vi "AlliGator Build Dataset Information String.vi"() -> (3 "Dataset Information String":string)   [LabVIEW 2021, in "AlliGator Dataset Information Window.lvlib"]
doc: "Creates <B>Dataset Information String</B> based on internal variables and settings."
uses:
  AlliGator Dataset Information Window.lvlib
  Globals, Variables, Constants/AlliGator Variables List.ctl
  Settings/AlliGator Settings List.ctl
  Variant/Variant to Data/Variant to String.vi
  Variant/Variant to Data/Variant to I32.vi
  Variant/Variant to Data/Variant to Boolean.vi
  Variant/Variant to Data/Variant to Path.vi
  Globals, Variables, Constants/AlliGator Globals, Variables & Constants.lvlib
  Variant/Variant to Data/Variant to Data.lvlib
  Settings/AlliGator Settings.lvlib
  Files/AlliGator Files.lvlib
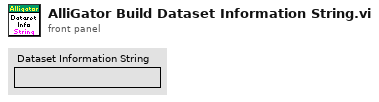
[diagram p1: front panel]
types:
  T1 = typedef "AlliGator Globals, Variables & Constants.lvlib/AlliGator Variables List.ctl" = enum16{"---- GUI ----", "GUI:Initialization Status", "GUI:State Indicators Refnum", "GUI:Original AlliGator Menu Items", "GUI:Current Action Loop State", "GUI:Script in progress", "GUI:Playback", "GUI:Loop Playback", "GUI:Search ROI Used", "GUI:Search ROI", "Decay Graph Max Legend Size", "Intensity Graph Max Legend Size", "Decay Statistics Graph Max Legend Size", "Phasor Graph Max Legend Size", "Phasor Ratio Graph Max Legend Size", "Lifetime Graph Max Legend Size", "---- Files ----", "Files:Export Dataset Frames as Individual Files", "Files:Show Batch Export Help Balloons", "Files:Frames in Dataset", "Files:ptu File Frame Start Indices", "Files:Current Frame in Dataset", "Files:Current Frame Timestamp", "Files:Dataset Loaded", "Files:Dataset Metadata", "Files:Dataset Channel", "Files:Dataset Data Description", "Files:Background Dataset Metadata", "Files:Background Dataset Channel", "Files:Background Dataset Data Description", "Files:Background File Subtraction", "Files:Background File Path", "Files:Background File Pile-up Correction", "Files:Background File Pixel Well Capacity", "Files:Background File Scaling Factor", "Files:Current Dataset Load Settings", "Files:Dataset Path", "Files:ICCD-specific Information", "Files:Macrotime Gate Separation", "------ Python Plugins ------", "Python Plugins:Information", "Python Plugins:Python Session", "Python Plugins:Valid Python Session?", "---- Source Image ----", "Source Image:ROIs", "Source Image:Current ROI", "Source Image:ROI Event Refnum", "X_Source Image Display Range", "X_Source Image Palette Information", "X_Type of Displayed Image", "X_Time Gate Slider", "Source Image:Palette List", "Source Image:Scale", "Source Image:ROI Overlay Color", "Source Image:Overlay to Erase", "Source Image:Is Displayed Image Accumulated", "Source Image:White Light Image Modified", "Source Image:Mask Image Modified", "---- Image Profile Window ----", "Image Profile:Window Event Refnum", "Image Profile:IntensityType", "Image Profile:Intensity Average Type", "Image Profile:Intensity-weighted SDV", "Image Profile:Box Profile Type", "Image Profile:Window Open", "Image Profile:Plotted Fit Parameter", "------ Phasor Graph -------", "Phasor Graph:Show Line", "---- Phasor Plot ---", "Phasor Plot:Parameters Changed", "Phasor Plot:FLI Dataset Modified since last Calculation", "Phasor Harmonics Data", "Selected Phasor Harmonics", "Phasor Harmonic Manager Event Refnum", "Phasor Plot:ROIs", "Phasor Plot:Current ROI", "Phasor Plot:ROI Event Refnum", "Phasor Plot:Image Reference Points", "Phasor Plot:Computed", "Phasor Plot:Palette Information", "Phasor Plot:Palette List", "Phasor Plot:Phasor Ratio Palette Information", "Phasor Plot:Phasor Ratio Palette List", "Phasor Plot:Image Scale", "Phasor Plot:Image Overlay to Erase", "Phasor Plot:Image Elements to Update", "Phasor Plot:Current Calculation Parameters", "Phasor Plot:Current Calibration Options", "Phasor Plot:Reset Cumulated Phasor Plot", "Phasor Plot:Reference 1", "Phasor Plot:Lifetime Reference 1", "Phasor Plot:Reference 1 Frequency", "Phasor Plot:Reference 2", "Phasor Plot:Lifetime Reference 2", "Phasor Plot:Reference 2 Frequency", "---- Decay Analysis ----", "Number of Selected Decays to Fit", "LS Fit Results", "LAR Fit Results", "BS Fit Results", "Last Decay Max - Min", "Best Fit Parameters", "Best Fit Parameter Names", "Actual Size X", "Actual Size Y", "Binning X", "Binning Y", "Actual # Gates", "Dataset Number", "Gates to...", "Gates Skipped", "Gates to keep", "Gate Step", "Gate Separation", "Reversed Gates", "Pile-up Correction", "Pixel Well Capacity", "Background Subtracted", "Background Subtraction Method", "Background Definition Range", "Background File (deprecated)", "Number of Dataset Accumulated", "Array of Accumulated Dataset Paths", "Do Averaged Datasets", "Destination File Path", "Process Plot Target", "Use 1/D as Phasor Frequency", "---- Decay Fit Parameter Map -----", "Decay Fit Parameter Map:Palette Information", "Decay Fit Parameter Map:Palette List", "---- Parameter Map ----", "Parameter Map:Palette Information", "Parameter Map:Palette List", "------- Local Decay Window ---------", "Local Decay Graph Window:Event Refnum", "Local Decay Graph Window:Use normalized IRF for convolution", "----- Miscellaneous ----", "Misc:Skippable Dialog Windows Status"}
  T2 = typedef "AlliGator Settings.lvlib/AlliGator Settings List.ctl" = enum16{"GUI:Visible Settings Tab", "GUI:Last Run Version", "Source Image:Use Image Histogram for Contrast", "Source Image:Low Count Pixels Rejection Options", "Source Image:High Count Pixels Rejection Options", "Source Image:Use Image Brightness", "Source Image:Blend Overlay with Image Background", "Source Image:Use Fixed ROI Diameter", "Source Image:ROI Diameter", "Source Image:ROI Center Color", "Source Image:Peak Threshold", "Source Image:Intensity Threshold", "Source Image:Image Binning Options", "Source Image:Image Smoothing Options", "Source Image:Image Histogram Active", "Source Image:Invert Binary Mask", "Source Image:Hot Pixel Removal", "Source Image:Overlay Analyzed ROI Center", "Source Image:Auto-Adjust Contrast", "Source Image:Histogram Lower Percentile", "Source Image:Histogram Upper Percentile", "Source Image:Save Source Image", "Source Image:Scale Bar Options", "Source Image:Image Resolution (Pixel Size)", "Source Image:Flatfield Correction", "Source Image:Show Dead Left Columns Correction", "Source Image:Dead Left Columns Correction", "Source Image:Image Pre-Processing Operations Order", "Source Image:Overlay ROI Median", "Source Image:Median Overlay Color", "Data Information:Gate Width", "Data Information:Nanotime Gate Separation", "Data Information:Macrotime Gate Separation", "Data Information:Gate Step", "Data Information:# Gates", "Data Information:Gate Image Exposure", "Data Information:Gate Image Integration", "Data Information:Gates to Skip", "Data Information:Gates to Keep", "Data Information:Define Gates to", "Data Information:Channel Name", "Data Information:Available Channel Names", "Data Information:Channel Arithmetic", "Data Information:Background File Subtraction", "Data Information:Background File", "Data Information:Background Scaling Factor", "Data Information:Background Pile-up Correction", "Data Information:Background Pixel Well Capacity", "Data Information:Laser Period", "Data Information:SYNC Period", "Data Information:Pile-up Correction", "Data Information:Pixel Well Capacity", "Data Information:Dataset Scaling Factor", "Fluorescence Decay_Decay Pre-Processing:Reverse Gates", "Fluorescence Decay_Decay Pre-Processing:Verbose Decay Pre-Processing", "Fluorescence Decay_Decay Pre-Processing:Use Decay Pre-Processing", "Fluorescence Decay_Decay Pre-Processing:Background Subtraction", "Fluorescence Decay_Decay Pre-Processing:Background Definition Range", "Fluorescence Decay_Decay Pre-Processing:Baseline Subtraction Method", "Fluorescence Decay_Decay Pre-Processing:Decay Pre-Processing Operations Order", "Fluorescence Decay_Decay Pre-Processing:Smoothing Parameter", "Fluorescence Decay_Decay Pre-Processing:Shift Decay", "Fluorescence Decay_Decay Pre-Processing:Decay Shift Parameters", "Fluorescence Decay_Decay Pre-Processing:Fold Decay", "Fluorescence Decay_Decay Pre-Processing:# Folds", "Fluorescence Decay_Decay Pre-Processing:1-Normalize Decay", "Fluorescence Decay_Decay Pre-Processing:[0-1]-Normalize Decay", "Fluorescence Decay_Decay Pre-Processing:Smoothen Decay", "Fluorescence Decay_Decay Pre-Processing:Extrapolate Decay", "Fluorescence Decay_Decay Pre-Processing:Use Periodicity", "Fluorescence Decay_Decay Pre-Processing:Use Cursors", "Fluorescence Decay_Decay Pre-Processing:Tail Fraction", "Fluorescence Decay_Decay Pre-Processing:Head Fraction", "Fluorescence Decay_Decay Pre-Processing:Additional Points", "Fluorescence Decay_Decay Pre-Processing:Straighten Decay", "Fluorescence Decay_Decay Pre-Processing:Constant Background", "Fluorescence Decay_Decay Pre-Processing:Pixel-Normalize Decay", "Fluorescence Decay_Advanced Analysis:Extract IRF instead of Decay", "Fluorescence Decay_Advanced Analysis:IRF Extraction Options", "Fluorescence Decay_Advanced Analysis:IRF Optimization Options", "Fluorescence Decay_Advanced Analysis:Square Pulse Options", "Fluorescence Decay_Advanced Analysis:IRF Order", "Fluorescence Decay_Advanced Analysis:IRF Time Constants", "Fluorescence Decay_Advanced Analysis:Wavelet Analysis Options", "Fluorescence Decay_Advanced Analysis:Average Lifetime Options", "Fluorescence Decay_Fit Options:Fit Options", "Fluorescence Decay_Fit Options:Use Legacy Fitting Approach", "Fluorescence Decay_Fit Options:Use Data Information Laser Period", "Fluorescence Decay_Fit Parameters:Displayed Fit Parameters", "Fluorescence Decay_Fit Parameters:Fit Parameter Constraints", "Fluorescence Decay_Fit Parameters:Export Tabulated Results", "Fluorescence Decay_Fit Parameters:MLE Baseline Offset Type", "Fluorescence Decay_Fit Parameters:MLE Baseline Offset", "Fluorescence Decay_Fit Parameters:Guess Parameter Names", "Fluorescence Decay_Fit Parameters:Guess Parameter Values", "Fluorescence Decay_Fit Parameters:Guess Parameters Options", "Fluorescence Decay_Styles:Show Last Decay Only", "Fluorescence Decay_Styles:Decay Graph Color Array", "Fluorescence Decay:Decay Graph Active", "Fluorescence Decay Statistics:Min Peak Value", "Fluorescence Decay Statistics:Reject Low Decay Peak Pixels", "Fluorescence Decay Statistics:Reject High Decay Peak Pixels", "Fluorescence Decay Statistics:Max Peak Value", "Time Traces:Use File Timestamp", "Time Traces:Time Step", "Time Traces:Use Intensity Correction File", "Time Traces:Intensity Correction File", "Phasor Plot:Phasor Plot Smoothing Options", "Phasor Plot:Phasor Plot Size", "Phasor Plot:Phasor Plot Graphics Options", "Phasor Plot:Cumulative Phasor Plot", "Phasor Plot:Use Phasor Brightness", "Phasor Plot:Blend Overlay with Phasor Background", "Phasor Plot:Save Phasor Plot", "Phasor Plot:Show References", "Phasor Plot:Phasor Ratio Decay Range", "Phasor Plot:Exponential Fading", "Phasor Plot:Phasor Ratio Reference Colors", "Phasor Plot:Reference Radius", "Phasor Plot:Show Color Map Vertices", "Phasor Plot:Phasor Plot Active", "Phasor Plot:Phasor Ratio Color Map Type", "Phasor Plot:Phasor Ratio Color Map", "Phasor Plot:Phasor Ratio Display Range", "Phasor Plot:Selected Image ROI(s)", "Phasor Plot:All Image ROIs", "Phasor Plot:Selected Phasor Plot ROI(s)", "Phasor Plot:All Phasor Plot ROIs", "Phasor Plot:Phasor Ratio Color-Coded Quantity", "Phasor Plot:Store Phasor Harmonics", "Phasor Plot:Draw Reference Segment", "Phasor Plot:User-Defined Quantity", "Phasor Graph:Phasor Frequency", "Phasor Graph:Phasor Ratio Type", "Phasor Graph:Pixel-level Phasor Computation", "Phasor Graph:Save Phasor Graph", "Phasor Graph:Phasor Graph Active", "Phasor Graph:Phasor SDV Options", "Phasor Calibration:Use Backup Calibration if needed", "Phasor Graph:Define Shortest Lifetime as", "Phasor Calibration:Backup Calibration Type", "Phasor Calibration:Calibration Type", "Phasor Calibration:Calibration Lifetime", "Phasor Calibration:Calibration Map Algorithm", "Single-Exponential Phasor Locus (SEPL):Gate Parameters", "Single-Exponential Phasor Locus (SEPL):User-defined Gate", "Single-Exponential Phasor Locus (SEPL):User-defined IRF", "Single-Exponential Phasor Locus (SEPL):Phasor Parameters", "Single-Exponential Phasor Locus (SEPL):Decay & IRF Parameters", "Single-Exponential Phasor Locus (SEPL):Display Parameters", "Lifetime Analysis:Decay Analysis Parameters", "Lifetime Analysis:Lifetime Map Active", "Plugins:Python Settings", "Miscellaneous:Verbose Mode", "Miscellaneous:Beep after Script", "Miscellaneous:Saved Image File Format", "Miscellaneous:Exported Gate Image Settings", "Miscellaneous:Include Loading in Timing", "Miscellaneous:Verbose Settings Mode", "Miscellaneous:Histogram Options", "Miscellaneous:Beep on Error", "Miscellaneous:# Logical Processors Used", "Miscellaneous:ROI Description Max Characters", "Miscellaneous:Verbose Error Mode", "Miscellaneous:Transparent Mask Color"}
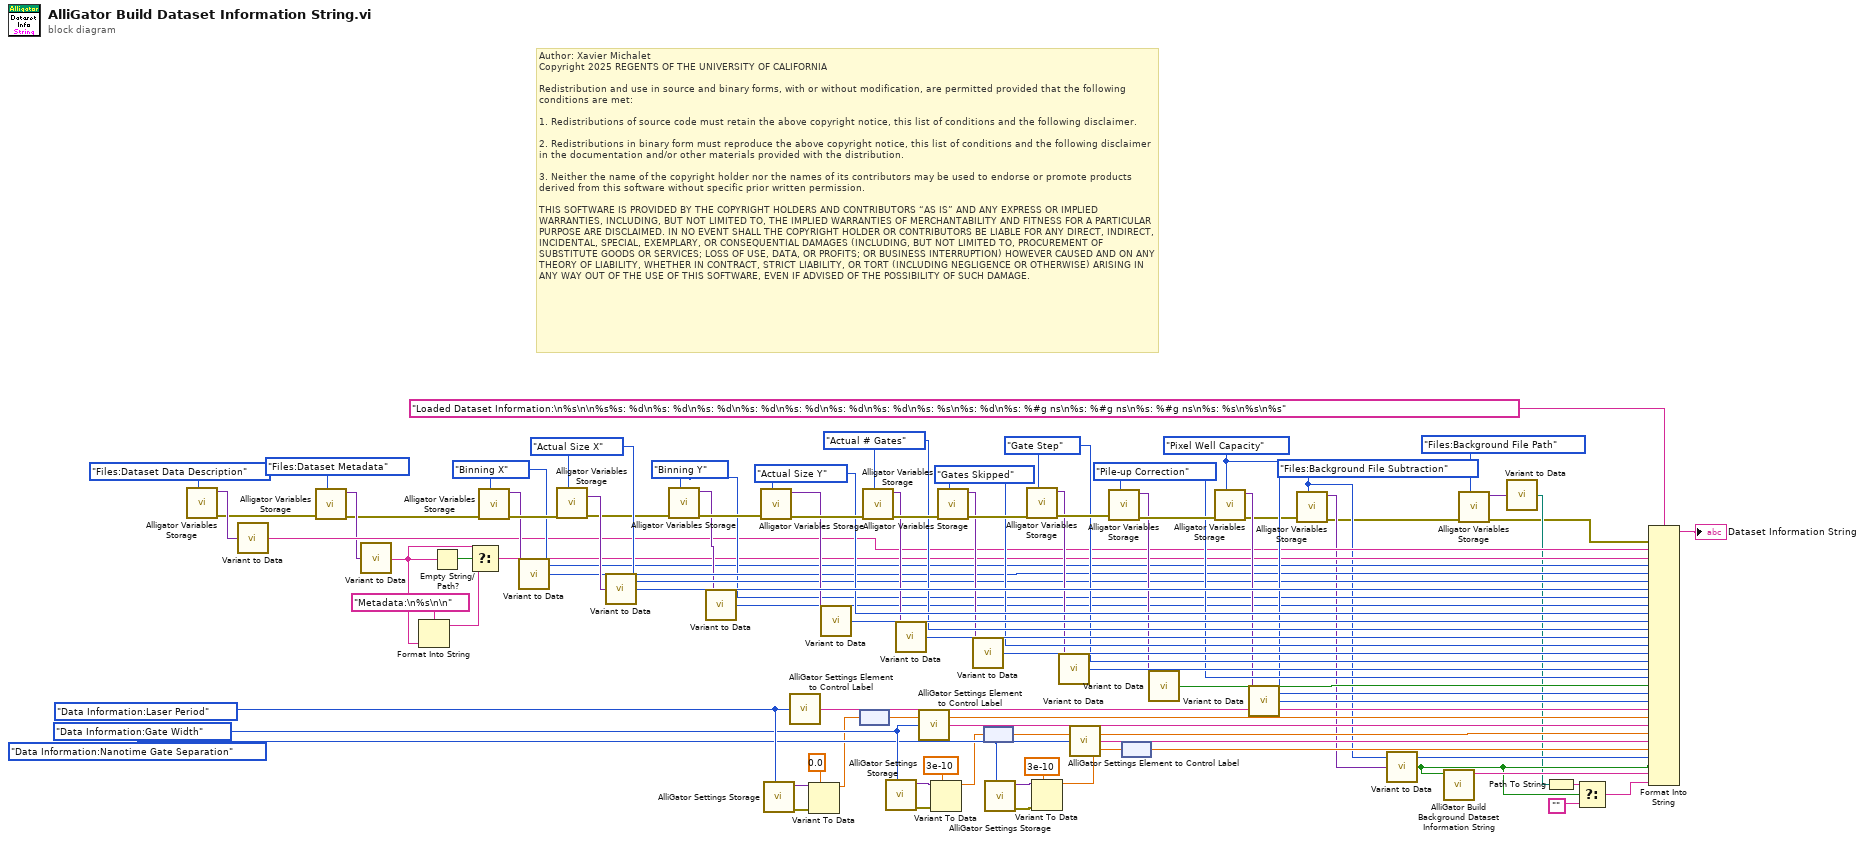
[diagram p0: block diagram]
diagram:
  w12 = AlliGator_Variables_List."Files:Background File Subtraction" ("Alligator Variable")
  w27 = AlliGator_Variables_List."Binning Y" ("Alligator Variable")
  w24 = AlliGator_Variables_List."Binning X" ("Alligator Variable")
  w46 = AlliGator_Settings_List."Data Information:Gate Width" ("AlliGator Settings List")
  w47 = AlliGator_Settings_List."Data Information:Laser Period" ("AlliGator Settings List")
  w45 = AlliGator_Settings_List."Data Information:Nanotime Gate Separation" ("AlliGator Settings List")
  w63 = AlliGator_Variables_List."Gate Step" ("Alligator Variable")
  w66 = AlliGator_Variables_List."Gates Skipped" ("Alligator Variable")
  w57 = AlliGator_Variables_List."Pixel Well Capacity" ("Alligator Variable")
  w60 = AlliGator_Variables_List."Pile-up Correction" ("Alligator Variable")
  w69 = AlliGator_Variables_List."Actual # Gates" ("Alligator Variable")
  w72 = AlliGator_Variables_List."Actual Size Y" ("Alligator Variable")
  w32 = AlliGator_Variables_List."Actual Size X" ("Alligator Variable")
  # "Author: Xavier Michalet\nCopyright 2025 REGENTS OF THE UNIVERSITY OF CALIFORNIA\n\nRedistribution and use in source and binary forms, with or without modification, are permitted provided that the following conditions are met:\n\n1. Redistributions of source code must retain the above copyright notice, this list of conditions and the following disclaimer.\n\n2. Redistributions in binary form must reproduce the above copyright notice, this list of conditions and the following disclaimer in the documentation and/or other materials provided with the distribution.\n\n3. Neither the name of the copyright holder nor the names of its contributors may be used to endorse or promote products derived from this software without specific prior written permission.\n\nTHIS SOFTWARE IS PROVIDED BY THE COPYRIGHT HOLDERS AND CONTRIBUTORS “AS IS” AND ANY EXPRESS OR IMPLIED WARRANTIES, INCLUDING, BUT NOT LIMITED TO, THE IMPLIED WARRANTIES OF MERCHANTABILITY AND FITNESS FOR A PARTICULAR PURPOSE ARE DISCLAIMED. IN NO EVENT SHALL THE COPYRIGHT HOLDER OR CONTRIBUTORS BE LIABLE FOR ANY DIRECT, INDIRECT, INCIDENTAL, SPECIAL, EXEMPLARY, OR CONSEQUENTIAL DAMAGES (INCLUDING, BUT NOT LIMITED TO, PROCUREMENT OF SUBSTITUTE GOODS OR SERVICES; LOSS OF USE, DATA, OR PROFITS; OR BUSINESS INTERRUPTION) HOWEVER CAUSED AND ON ANY THEORY OF LIABILITY, WHETHER IN CONTRACT, STRICT LIABILITY, OR TORT (INCLUDING NEGLIGENCE OR OTHERWISE) ARISING IN ANY WAY OUT OF THE USE OF THIS SOFTWARE, EVEN IF ADVISED OF THE POSSIBILITY OF SUCH DAMAGE."
  n1 = call "Alligator Variables Storage.vi"("AlliGator Variable"=AlliGator_Variables_List."Files:Dataset Data Description" ("Alligator Variable")) -> ("Error Out"=w20:errorcluster, "Data out"=w82:variant)  [unwired: 8 in, 1 out]
  n2 = call-poly "Variant to Data.vi"("Variant"=w82) -> ("String"=w23:string)  [unwired: 8 in]
  n3 = call "Alligator Variables Storage.vi"("AlliGator Variable"=AlliGator_Variables_List."Files:Dataset Metadata" ("Alligator Variable"), "Error In"=w20) -> ("Error Out"=w19:errorcluster, "Data out"=w22:variant)  [unwired: 7 in, 1 out]
  n4 = call-poly "Variant to Data.vi"("Variant"=w22) -> ("String"=w15:string)  [unwired: 8 in]
  n5 = Format Into String(format string="Metadata:\n%s\n\n", w15) -> (resulting string=w16:string)  [unwired: 2 in, 1 out]
  n6 = Empty String/Path?(string/path=w15) -> (empty?=w18:bool)
  n7 = Select(t=w15, s=w18, f=w16) -> (s? t:f=w17:string)
  n8 = call "Alligator Variables Storage.vi"("AlliGator Variable"=w24, "Error In"=w19) -> ("Error Out"=w33:errorcluster, "Data out"=w31:variant)  [unwired: 7 in, 1 out]
  n9 = call-poly "Variant to Data.vi"("Variant"=w31) -> ("Value"=w30:i32)  [unwired: 8 in]
  n10 = call "Alligator Variables Storage.vi"("AlliGator Variable"=w32, "Error In"=w33) -> ("Error Out"=w29:errorcluster, "Data out"=w74:variant)  [unwired: 7 in, 1 out]
  n11 = call-poly "Variant to Data.vi"("Variant"=w74) -> ("Value"=w73:i32)  [unwired: 8 in]
  n12 = call "Alligator Variables Storage.vi"("AlliGator Variable"=w27, "Error In"=w29) -> ("Error Out"=w28:errorcluster, "Data out"=w26:variant)  [unwired: 7 in, 1 out]
  n13 = call-poly "Variant to Data.vi"("Variant"=w26) -> ("Value"=w25:i32)  [unwired: 8 in]
  n14 = call "Alligator Variables Storage.vi"("AlliGator Variable"=w72, "Error In"=w28) -> ("Error Out"=w76:errorcluster, "Data out"=w71:variant)  [unwired: 7 in, 1 out]
  n15 = call "AlliGator Settings Storage.vi"("AlliGator Settings List"=w47) -> ("Error Out"=w53:errorcluster, "Variant Data out"=w54:variant)  [unwired: 9 in]
  n16 = call "AlliGator Settings Element to Control Label.vi"("AlliGator Settings List"=w47) -> ("Label"=w43:string)  [unwired: 8 in]
  n17 = Variant To Data(error in=w53, type=dbl[unit] 0.0 ("Laser Period"), Variant=w54) -> (data=w42:dbl[unit])  [unwired: 1 out]
  n18 = call-poly "Variant to Data.vi"("Variant"=w71) -> ("Value"=w70:i32)  [unwired: 8 in]
  n19 = node(w42) -> (w41:dbl)
  n20 = call "Alligator Variables Storage.vi"("AlliGator Variable"=w69, "Error In"=w76) -> ("Error Out"=w78:errorcluster, "Data out"=w68:variant)  [unwired: 7 in, 1 out]
  n21 = call "AlliGator Settings Storage.vi"("AlliGator Settings List"=w46) -> ("Error Out"=w51:errorcluster, "Variant Data out"=w52:variant)  [unwired: 9 in]
  n22 = call-poly "Variant to Data.vi"("Variant"=w68) -> ("Value"=w67:i32)  [unwired: 8 in]
  n23 = call "AlliGator Settings Element to Control Label.vi"("AlliGator Settings List"=w46) -> ("Label"=w40:string)  [unwired: 8 in]
  n24 = Variant To Data(error in=w51, type=dbl[unit] 3e-10 ("Gate Duration"), Variant=w52) -> (data=w39:dbl[unit])  [unwired: 1 out]
  n25 = call "Alligator Variables Storage.vi"("AlliGator Variable"=w66, "Error In"=w78) -> ("Error Out"=w79:errorcluster, "Data out"=w65:variant)  [unwired: 7 in, 1 out]
  n26 = call-poly "Variant to Data.vi"("Variant"=w65) -> ("Value"=w64:i32)  [unwired: 8 in]
  n27 = node(w39) -> (w38:dbl)
  n28 = call "AlliGator Settings Storage.vi"("AlliGator Settings List"=w45) -> ("Error Out"=w49:errorcluster, "Variant Data out"=w50:variant)  [unwired: 9 in]
  n29 = call "Alligator Variables Storage.vi"("AlliGator Variable"=w63, "Error In"=w79) -> ("Error Out"=w80:errorcluster, "Data out"=w62:variant)  [unwired: 7 in, 1 out]
  n30 = Variant To Data(error in=w49, type=dbl[unit] 3e-10 ("Gate Duration"), Variant=w50) -> (data=w35:dbl[unit])  [unwired: 1 out]
  n31 = call-poly "Variant to Data.vi"("Variant"=w62) -> ("Value"=w61:i32)  [unwired: 8 in]
  n32 = call "AlliGator Settings Element to Control Label.vi"("AlliGator Settings List"=w45) -> ("Label"=w37:string)  [unwired: 8 in]
  n33 = call "Alligator Variables Storage.vi"("AlliGator Variable"=w60, "Error In"=w80) -> ("Error Out"=w77:errorcluster, "Data out"=w59:variant)  [unwired: 7 in, 1 out]
  n34 = node(w35) -> (w34:dbl)
  n35 = call-poly "Variant to Data.vi"("Variant"=w59) -> ("Value"=w58:bool)  [unwired: 8 in]
  n36 = call "Alligator Variables Storage.vi"("AlliGator Variable"=w57, "Error In"=w77) -> ("Error Out"=w13:errorcluster, "Data out"=w55:variant)  [unwired: 7 in, 1 out]
  n37 = call-poly "Variant to Data.vi"("Variant"=w55) -> ("Value"=w56:i32)  [unwired: 8 in]
  n38 = call "Alligator Variables Storage.vi"("AlliGator Variable"=w12, "Error In"=w13) -> ("Error Out"=w9:errorcluster, "Data out"=w11:variant)  [unwired: 7 in, 1 out]
  n39 = call-poly "Variant to Data.vi"("Variant"=w11) -> ("Value"=w6:bool)  [unwired: 8 in]
  n40 = call "AlliGator Build Background Dataset Information String.vi"("Bkgd Subtraction"=w6) -> ("Background Dataset Description"=w10:string)  [unwired: 9 in, 1 out]
  n41 = call "Alligator Variables Storage.vi"("AlliGator Variable"=AlliGator_Variables_List."Files:Background File Path" ("Alligator Variable"), "Error In"=w9) -> ("Error Out"=w1:errorcluster, "Data out"=w7:variant)  [unwired: 7 in, 1 out]
  n42 = call-poly "Variant to Data.vi"("Variant"=w7) -> ("Path"=w5:path)  [unwired: 8 in]
  n43 = Path To String(path=w5) -> (string=w3:string)
  n44 = Select(t=w3, s=w6, f="") -> (s? t:f=w4:string)
  n45 = Format Into String(format string="Loaded Dataset Information:\n%s\n\n%s%s: %d\n%s: %d\n%s: %d\n%s: %d\n%s: %d\n%s: %d\n%s: %d\n%s: %s\n%s: %d\n%s: %#g ns\n%s: %#g ns\n%s: %#g ns\n%s: %s\n%s\n%s", error in=w1, w23, w17, w24, w30, w32, w73, w27, w25, w72, w70, w69, w67, w66, w64, w63, w61, w60, w58, w57, w56, w43, w41, w40, w38, w37, w34, w12, w6, w10, w4) -> (resulting string=→"Dataset Information String":string)  [unwired: 1 in, 1 out]
